vi "RunM100Recipe.vi"   [LabVIEW 2012]
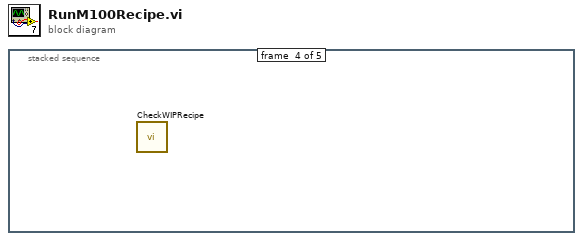
[diagram p0: block diagram]
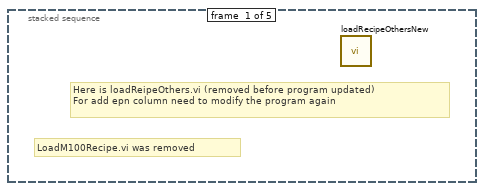
[diagram p2: hidden frame]
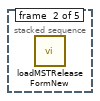
[diagram p3: hidden frame]
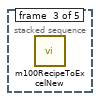
[diagram p4: hidden frame]
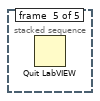
[diagram p5: hidden frame]
diagram:
  n1 = stacked-sequence {
    frame #0 {
      # "Here is loadReipeOthers.vi (removed before program updated)\nFor add epn column need to modify the program again"
      # "LoadM100Recipe.vi was removed"
      n2 = call "loadRecipeOthersNew.vi"() -> ()  [unwired: 12 in]
    }
    frame #1 {
      n3 = call "loadMSTReleaseFormNew.vi"() -> ()  [unwired: 12 in]
    }
    frame #2 {
      n4 = call "m100RecipeToExcelNew.vi"() -> ()  [unwired: 12 in]
    }
    frame #3 {
      n5 = call "CheckWIPRecipe.vi"() -> ()  [unwired: 12 in]
    }
    frame #4 {
      n6 = Quit LabVIEW() -> ()  [unwired: 1 in]
    }
  }
